vi "Array_filter_elements.vi"(10 "smaller set":dbl[](array[numeric])=[0.0, 0.0, 1.0, 3.0], 11 "larger set":dbl[](array[numeric])=[3.0, 3.0, 3.0, 4.0, 5.0, 0.0]) -> (1 "shared":dbl[](array[numeric])=[0.0, 0.0, 0.0, 3.0], 2 "deleted":dbl[](array[numeric])=[0.0, 1.0], 3 "filtered":dbl[](array[numeric])=[3.0, 3.0, 4.0, 5.0])   [LabVIEW 2020]
panel:
  # "Compare two 1D arrays\nFiltered: Elements present in both smaller and larger sets are deleted from the larger set"
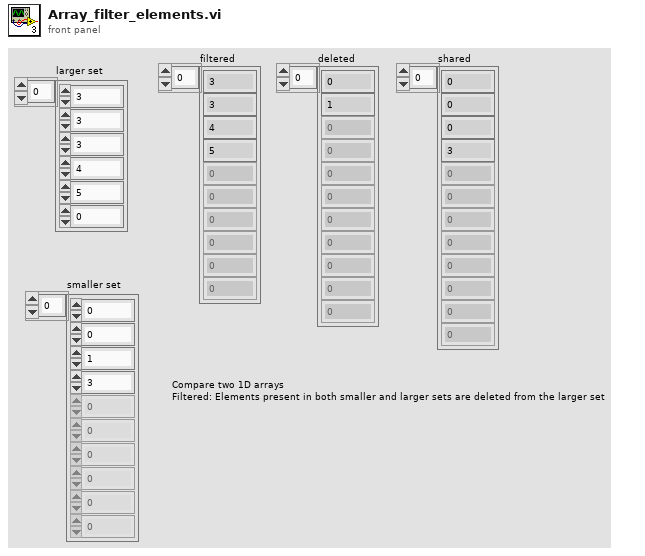
[diagram p1: front panel]
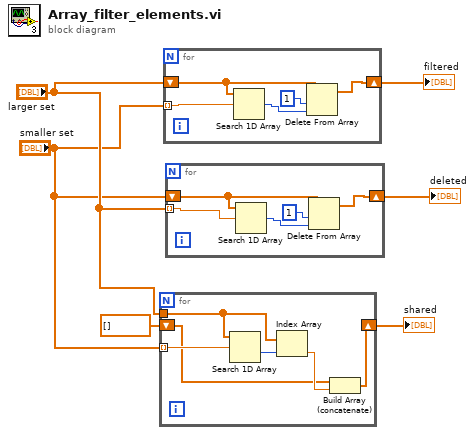
[diagram p0: block diagram]
diagram:
  n1 = for {
    shift-right: [w8] -> w1
    shift-left: dbl[] [] -> [w7]
    tunnel: "larger set" -> [w11]
    tunnel: "smaller set" -> [w12] mode=indexing
    n2 = Search 1D Array(1D array=w11, element=w12) -> (index of element=w10:i32)  [unwired: 1 in]
    n3 = Index Array(array=w11, index=w10) -> (element=w9:dbl)
    n4 = Build Array (concatenate)(w7, w9) -> (w8:dbl[])
  }
  "shared" <- w1
  n5 = for {
    tunnel: "smaller set" -> [w17] mode=indexing
    shift-right: [w13] -> w6
    shift-left: "larger set" -> [w16]
    n6 = Search 1D Array(1D array=w16, element=w17) -> (index of element=w15:i32)  [unwired: 1 in]
    n7 = Delete From Array(array=w16, length=1, index=w15) -> (array with subset deleted=w13:dbl[])  [unwired: 1 out]
  }
  "filtered" <- w6
  n8 = for {
    tunnel: "larger set" -> [w22] mode=indexing
    shift-right: [w18] -> w5
    shift-left: "smaller set" -> [w21]
    n9 = Search 1D Array(1D array=w21, element=w22) -> (index of element=w20:i32)  [unwired: 1 in]
    n10 = Delete From Array(array=w21, length=1, index=w20) -> (array with subset deleted=w18:dbl[])  [unwired: 1 out]
  }
  "deleted" <- w5
